vi "LogDBIntChange.vi"(6 "current time":timestamp, 7 "db table name":string, 8 "error in":errorcluster, 9 "value":u32, 10 "shiftReg":u32, 11 "Refnum in":T1) -> (0 "error out":errorcluster, 2 "shiftReg":u32, 3 "Refnum out":T1)   [LabVIEW 2011]
uses:
  <vilib>/addons/database/Connection.llb/Conn ObjectReference.ctl
  <vilib>/addons/database/NI_Database_API.lvlib
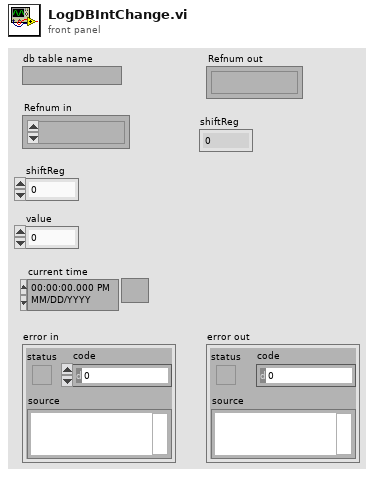
[diagram p1: front panel]
types:
  T1 = typedef "NI_Database_API.lvlib/Conn ObjectReference.ctl" = refnum<k1>
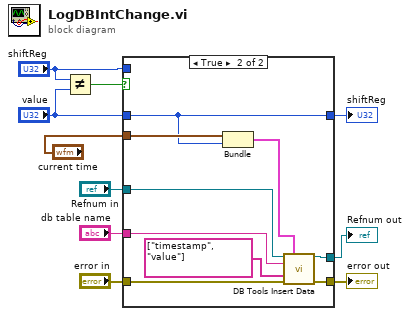
[diagram p0: block diagram]
diagram:
  n1 = Not Equal?(x="shiftReg", y="value") -> (x != y?=w4:bool)
  n2 = case shown="True" w4 {
    tunnel: [w11 w14] -> w8
    tunnel: [w13 w20] -> w7
    tunnel: "Refnum in" -> [w13 w21]
    tunnel: "db table name" -> [_ w22]
    tunnel: "error in" -> [w12 w19]
    tunnel: [w12 w18] -> w10
    tunnel: "current time" -> [_ w17]
    tunnel: "value" -> [_ w14]
    tunnel: "shiftReg" -> [w11 _]
    frame False {
    }
    frame True {
      n3 = Bundle("current time"=w17, "value"=w14) -> (w16:cluster{"current time":timestamp, "value":u32})  [unwired: 1 in]
      n4 = call <vilib>:"DB Tools Insert Data.vi"("connection reference"=w21, "data"=w16, "table"=w22, "columns"=string[] ["timestamp", "value"], "error in (no error)"=w19) -> ("connection reference out"=w20:T1, "error out"=w18:errorcluster)  [unwired: 9 in]
    }
  }
  "error out" <- w10
  "shiftReg" <- w8
  "Refnum out" <- w7
